vi "Termistor y motor.vi"() -> ()   [LabVIEW 2017]
uses:
  <vilib>/LabVIEW Interface for Arduino/Type Defs/Analog Pin.ctl
  <vilib>/LabVIEW Interface for Arduino/LabVIEW Interface for Arduino.lvlib
panel:
  out "output variable":dbl
  out "WAVE TEMP":dbl(graph)
  out "TEMP GAUGE":dbl(slide) scale=0.0..100.0
  out "Voltage":dbl(knob) scale=0.0..5.0
  in  "Stop":bool
  in  "Analog Pin":T1
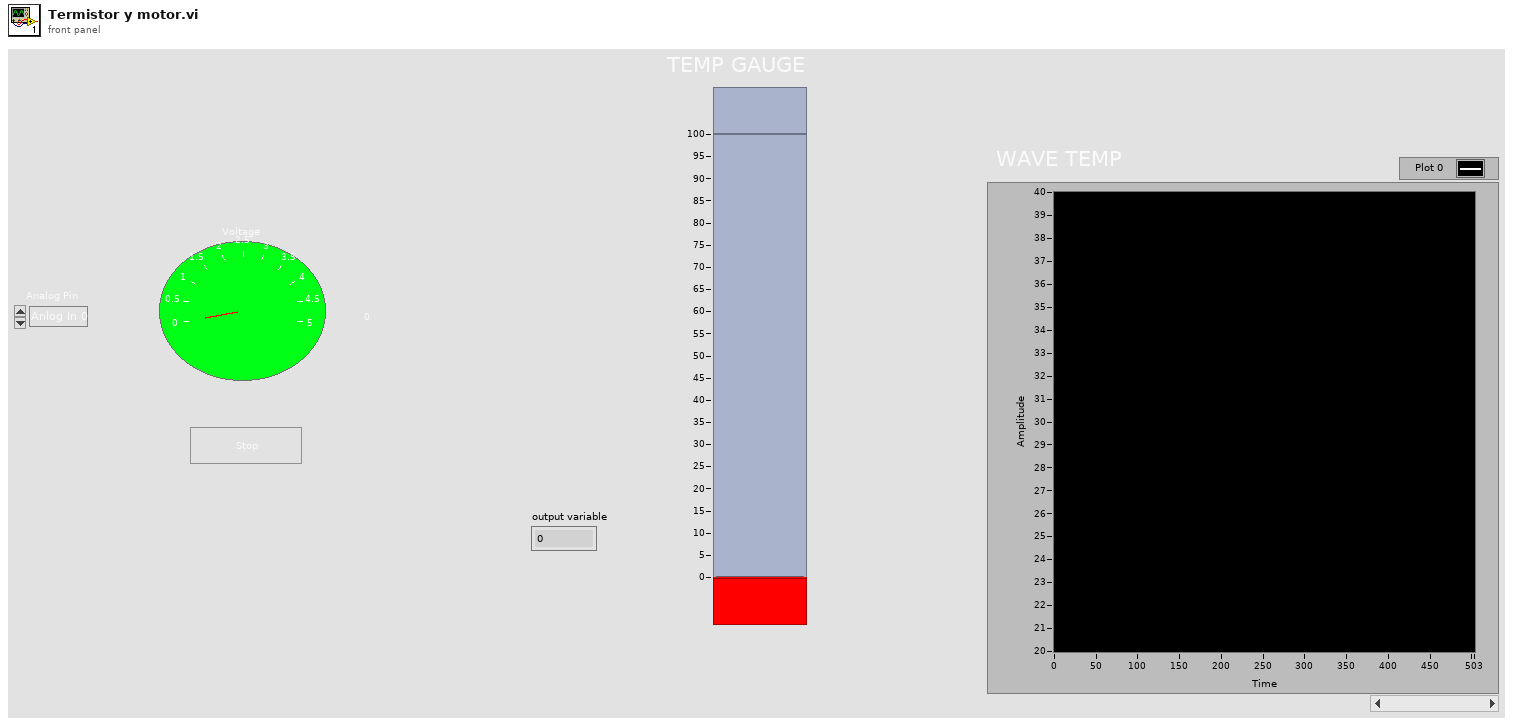
[diagram p1: front panel]
types:
  T1 = typedef "LabVIEW Interface for Arduino.lvlib/Analog Pin.ctl" = enum8{"Anlog In 0", "Anlog In 1", "Anlog In 2", "Anlog In 3", "Anlog In 4", "Anlog In 5"}
  T2 = typedef "LabVIEW Interface for Arduino.lvlib/Arduino Resource.ctl" = cluster{"VISA resource":refnum<visa-resource-name>, "Board Type":T3, "Connection Type":enum8{"USB / Serial"}, "Bytes Per Packet (15)":u8}
  T3 = typedef "LabVIEW Interface for Arduino.lvlib/Board Type.ctl" = enum16{"Uno", "Dimuelanove w/Atmega 328", "Mega 2560"}
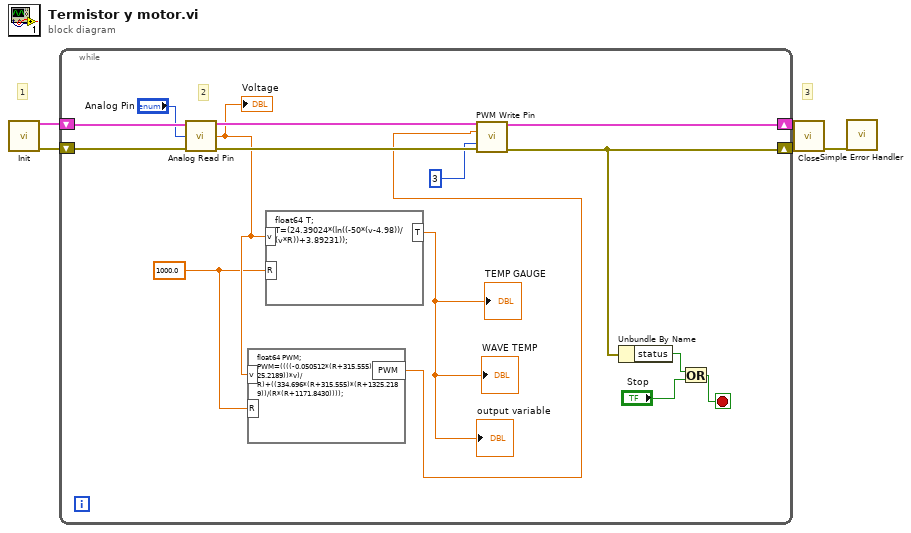
[diagram p0: block diagram]
diagram:
  # "3"
  # "1"
  n1 = call <vilib>:"Init.vi"() -> ("Arduino Resource"=w5:T2, "error out"=w2:errorcluster)  [unwired: 18 in]
  n2 = while {
    shift-right: [w13] -> w4
    shift-left: w5 -> [w17]
    shift-right: [w6] -> w3
    shift-left: w2 -> [w16]
    stop <- w20 stop-if-true
    w8 = 1000.0 ("input variable")
    # "2"
    n3 = call <vilib>:"Analog Read Pin.vi"("Arduino Resource"=w17, "Analog Input Pin (0)"="Analog Pin", "error in"=w16) -> ("Arduino Resource"=w14:T2, "Voltage"=w9:dbl, "error out"=w12:errorcluster)  [unwired: 10 in]
    "Voltage" <- w9
    n4 = formula code="float64 PWM;\nPWM=((((-0.050512*(R+315.555)*(R+1325.2189))*v)/R)+((334.696*(R+315.555)*(R+1325.2189))/(R*(R+1171.8430))));"("v"=w9, "R"=w8) -> ("PWM"=w7:dbl)
    n5 = formula code="float64 T;\nT=(24.39024*(ln((-50*(v-4.98))/(v*R))+3.89231));"("v"=w9, "R"=w8) -> ("T"=→"TEMP GAUGE" →"WAVE TEMP" →"output variable":dbl)
    n6 = call <vilib>:"PWM Write Pin.vi"("Arduino Resource"=w14, "Duty Cycle (0 - 255)"=w7, "PWM Pin (3)"=u8 3, "error in"=w12) -> ("Arduino Resource"=w13:T2, "error out"=w6:errorcluster)  [unwired: 10 in]
    n7 = Unbundle By Name(w6) -> ("status"=w19:bool)
    n8 = Or(x=w19, y="Stop") -> (x .or. y?=w20:bool)
  }
  n9 = call <vilib>:"Close.vi"("Arduino Resource"=w4, "error in"=w3) -> ("error out"=w1:errorcluster)  [unwired: 13 in]
  n10 = call <vilib>:"Simple Error Handler.vi"("error in (no error)"=w1) -> ()  [unwired: 4 in, 5 out]
